vi "Stop Core.vi"(10 "final error code":i32, 11 "Assert Startup UI in":refnum<class "Assert Startup UI.lvclass">) -> (3 "Assert Startup UI out":refnum<class "Assert Startup UI.lvclass">)   [LabVIEW 2016, in "Assert API Components.lvlib" / "Assert Startup UI.lvlib" / "Assert Startup UI.lvclass"]
doc: "(<B>Filename</B>: Actor Framework.lvlib:Actor.lvclass:Stop Core.vi)\n\nDefines what the actor does before it stops. Use the <B>final error code</B> input to determine whether the actor shut down in response to an error.\n\nBy default, this method does nothing. A descendant class may override it to define behavior, such as shutting down any processes the actor initiated in its override of the Actor Core method."
uses:
  Assert Startup UI.lvclass
  Assert Startup UI.lvclass/Assert Startup UI.ctl
  Base UI Actor/Base UI Actor/Base UI Actor.lvclass
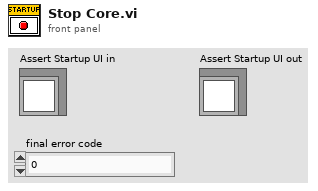
[diagram p1: front panel]
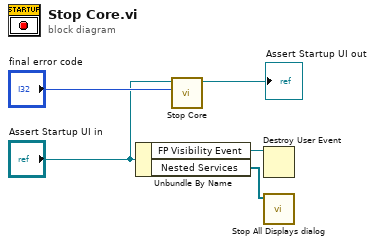
[diagram p0: block diagram]
diagram:
  n1 = Unbundle By Name("Assert Startup UI in") -> ("FP Visibility Event"=w1:refnum<user-event>, "Nested Services"=w2:refnum<class "Message Enqueuer.lvclass">[])
  n2 = call-parent "Stop Core.vi"("final error code"="final error code", "Base UI Actor in"="Assert Startup UI in") -> ("Base UI Actor out"=→"Assert Startup UI out":refnum<class "Assert Startup UI.lvclass">)  [unwired: 9 in]
  n3 = Destroy User Event(user event=w1) -> ()  [unwired: 1 in, 1 out]
  n4 = call "Stop All Displays dialog.vi"("Displays"=w2) -> ()  [unwired: 11 in]
